vi "U3 eAIN Loop with Chart .vi"() -> (0 "error out":errorcluster)   [LabVIEW 2018]
panel:
  out "Waveform Chart":dbl(graph)
  in  "stop":bool
  in  "Interval (ms)":u32=500
  in  "FirstFound":bool=TRUE
  in  "Address":string="1"
  out "Error Message":string
  out "AIN0 Voltage":dbl format="%.6f"
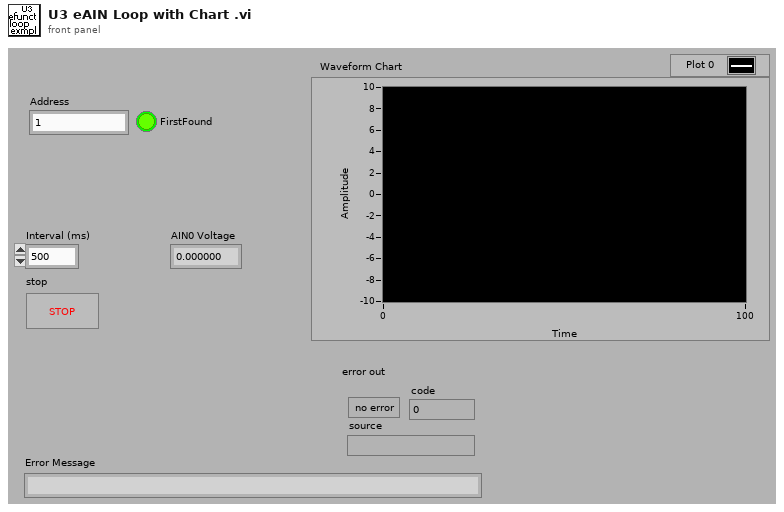
[diagram p1: front panel]
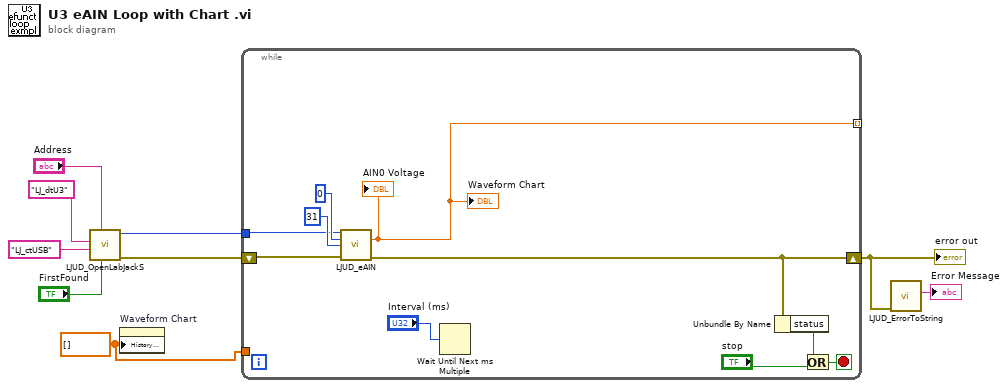
[diagram p0: block diagram]
diagram:
  w1 = dbl[] [] ("History Data")
  n1 = call "LJUD_OpenLabJackS.vi"("FirstFound"="FirstFound", "Address"="Address", "ConnectionType"="LJ_ctUSB", "DeviceType"="LJ_dtU3") -> ("error out"=w2:errorcluster, "Handle"=w4:i32)  [unwired: 5 in, 1 out]
  n2 = property on="Waveform Chart" class="WFChart (strict)"("History Data"=w1) -> ()  [unwired: 2 in, 2 out]
  n3 = while {
    shift-left: w2 -> [w13]
    shift-right: [w11] -> w3
    tunnel: w4 -> [w12]
    tunnel: w1 -> [_]
    tunnel: [w10] -> _ mode=indexing
    stop <- w16 stop-if-true
    n4 = call "LJUD_eAIN.vi"("Handle In"=w12, "ChannelP"=0, "ChannelN"=31, "error in"=w13) -> ("Voltage"=w10:dbl, "error out"=w11:errorcluster)  [unwired: 9 in, 1 out]
    "AIN0 Voltage" <- w10
    "Waveform Chart" <- w10
    n5 = Wait Until Next ms Multiple(millisecond multiple="Interval (ms)") -> ()  [unwired: 1 out]
    n6 = Unbundle By Name(w11) -> ("status"=w15:bool)
    n7 = Or(x=w15, y="stop") -> (x .or. y?=w16:bool)
  }
  "error out" <- w3
  n8 = call "LJUD_ErrorToString.vi"("error in"=w3) -> ("String"=→"Error Message":string)  [unwired: 10 in]
